vi "Send Command - Reset.vi"(0 "VISA resource name":refnum<visa-resource-name>, 11 "error in (no error)":errorcluster) -> (4 "VISA resource name out":refnum<visa-resource-name>, 15 "error out":errorcluster)   [LabVIEW 2020, in "Associated Research 78XX Series.lvlib"]
doc: "RESET\nStop or abort a test. Also used to reset a latched failure condition."
uses:
  <instrlib>/Associated Research 78XX Series/Associated Research 78XX Series.lvlib
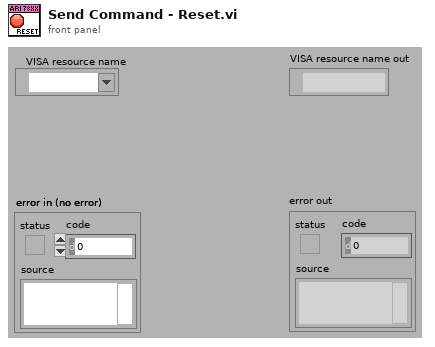
[diagram p1: front panel]
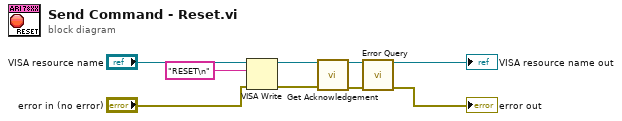
[diagram p0: block diagram]
diagram:
  n1 = VISA Write(VISA resource name="VISA resource name", write buffer="RESET\n" ("\"False\" Command"), error in (no error)="error in (no error)") -> (VISA resource name out=w3:refnum<visa-resource-name>, error out=w4:errorcluster)  [unwired: 1 out]
  n2 = call <instrlib>:"Get Acknowledgement.vi"("VISA resource name"=w3, "error in (no error)"=w4) -> ("VISA resource name out"=w7:refnum<visa-resource-name>, "error out"=w5:errorcluster)  [unwired: 12 in]
  n3 = call <instrlib>:"Error Query.vi"("VISA resource name"=w7, "error in (no error)"=w5) -> ("VISA resource name out"=→"VISA resource name out":refnum<visa-resource-name>, "error out"=→"error out":errorcluster)  [unwired: 10 in, 2 out]
